vi "RSNRPZ Add Sensor.vi"(6 "Channel (2)":i32=2, 7 "Resource Name (USB::0xaad::0x00b::100000)":string="USB::0xaad::0x00b::100000", 8 "error in (no error)":errorcluster, 9 "Reset Device (T: Reset Device)":bool=TRUE, 10 "ID Query (T: Do Query)":bool=TRUE, 11 "VISA session":refnum<visa-resource-name> caption="VISA resource name") -> (0 "error out":errorcluster, 3 "dup VISA session":refnum<visa-resource-name> caption="VISA resource name")   [LabVIEW 2010]
doc: "This VI performs the following initialization actions and adds sensor to channel list:\n\n- Opens a session to the specified device using the interface and address specified in the Resource Name control.\n\n- Performs an identification query on the Instrument.\n\n- Resets the instrument to a known state.\n\n- Sends initialization commands to the sensor"
uses:
  rsnrpz_32.dll
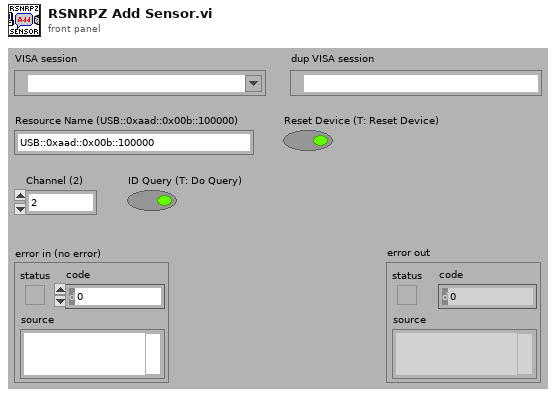
[diagram p1: front panel]
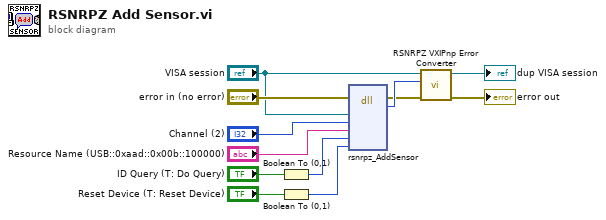
[diagram p0: block diagram]
diagram:
  n1 = Boolean To (0,1)(Boolean="ID Query (T: Do Query)") -> (0, 1=w7:i16)
  n2 = Boolean To (0,1)(Boolean="Reset Device (T: Reset Device)") -> (0, 1=w6:i16)
  n3 = dll-call lib="rsnrpz_32.dll" fn="rsnrpz_AddSensor"(error in="error in (no error)", "Instrument Handle"="VISA session", "Channel"="Channel (2)", "Resource Name"="Resource Name (USB::0xaad::0x00b::100000)", "ID Query"=w7, "Reset Device"=w6) -> (error out=w5:errorcluster, "Status"=w10:i32)  [unwired: 7 in, 1 out]
  n4 = call <instrlib>:"RSNRPZ VXIPnp Error Converter.vi"("error in"=w5, "VXIPnp error code"=w10, "VISA session"="VISA session") -> ("error out"=→"error out":errorcluster, "dup VISA session"=→"dup VISA session":refnum<visa-resource-name>)  [unwired: 7 in]
